vi "Update Step Start Timestamp.vi"(8 "error in (no error)":errorcluster, 9 "Previous step end timestamp":dbl, 10 "Current Time":timestamp, 11 "Output Sequencer in":refnum<class "Output Sequencer.lvclass">) -> (0 "error out":errorcluster, 3 "Output Sequencer out":refnum<class "Output Sequencer.lvclass">)   [LabVIEW 2020, in "Output Sequencer.lvlib" / "Output Sequencer.lvclass"]
uses:
  Output Sequencer.lvclass
  Output Sequencer.lvclass/Output Sequencer.ctl
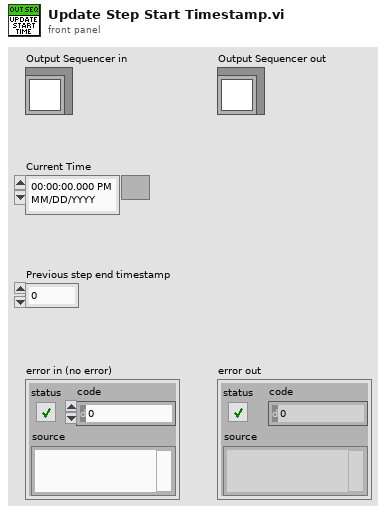
[diagram p1: front panel]
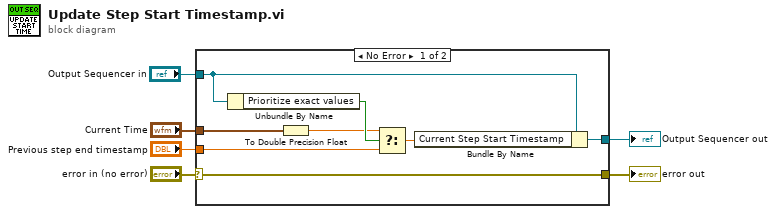
[diagram p0: block diagram]
diagram:
  n1 = case shown="No Error" "error in (no error)" {
    selector: "error in (no error)" -> [w7 w15]
    tunnel: [w14 w16] -> w6
    tunnel: "Previous step end timestamp" -> [w13 _]
    tunnel: "Current Time" -> [w12 _]
    tunnel: "Output Sequencer in" -> [w11 w16]
    tunnel: [w7 w15] -> w1
    frame No Error {
      n2 = Unbundle By Name(w11) -> ("Prioritize exact values"=w10:bool)
      n3 = To Double Precision Float(number=w12) -> (double precision float=w8:dbl)
      n4 = Select(t=w8, s=w10, f=w13) -> (s? t:f=w9:dbl)
      n5 = Bundle By Name(cluster=w11, "Current Step Start Timestamp"=w9) -> (w14:refnum<class "Output Sequencer.lvclass">)
    }
    frame Error {
    }
  }
  "Output Sequencer out" <- w6
  "error out" <- w1
